vi "Read Limiter Msg.vi"(8 "error in (no error)":errorcluster, 11 "Helm Limiter Msg in":refnum<class "Helm Limiter Msg.lvclass">) -> (0 "error out":errorcluster, 2 "Limiter":dbl, 3 "Helm Limiter Msg out":refnum<class "Helm Limiter Msg.lvclass">)   [LabVIEW 2015, in "RDS Child Messages.lvlib" / "Helm Limiter Msg.lvclass"]
uses:
  Helm Limiter Msg.lvclass
  Helm Limiter Msg.lvclass/Helm Limiter Msg.ctl
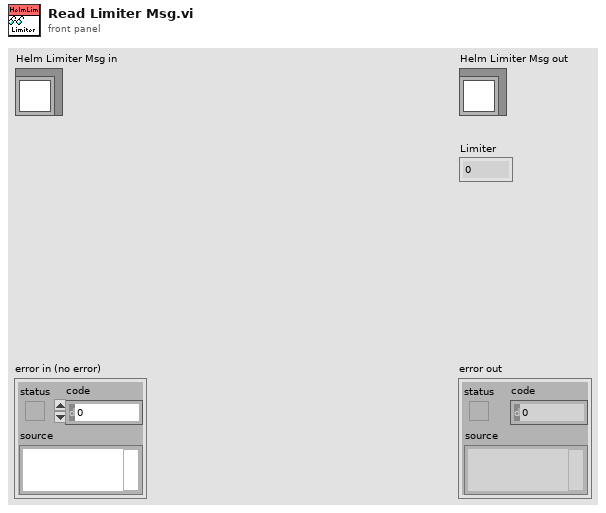
[diagram p1: front panel]
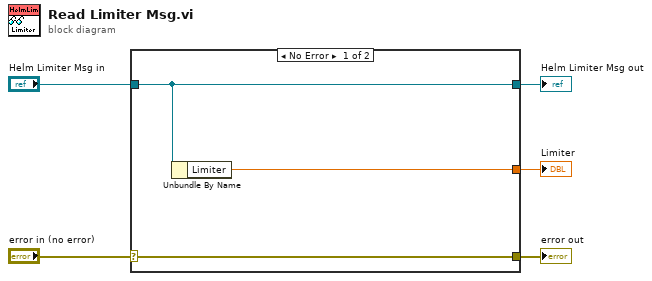
[diagram p0: block diagram]
diagram:
  n1 = case shown="No Error" "error in (no error)" {
    selector: "error in (no error)" -> [w8 w9]
    tunnel: [w8 w9] -> w4
    tunnel: [w7 w10] -> w2
    tunnel: "Helm Limiter Msg in" -> [w7 w10]
    tunnel: [w6 _] -> w1
    frame No Error {
      n2 = Unbundle By Name(w7) -> ("Limiter"=w6:dbl)
    }
    frame Error {
    }
  }
  "error out" <- w4
  "Helm Limiter Msg out" <- w2
  "Limiter" <- w1
